vi "Remove trailing zeros.vi"(11 "Number":string) -> (3 "Number with trainlg zeros removed":string)   [LabVIEW 2017, in "JSONtext.lvlib"]
uses:
  JSONtext.lvlib
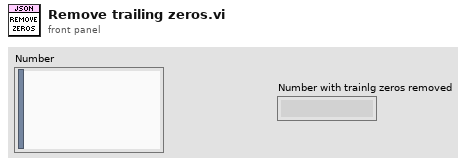
[diagram p1: front panel]
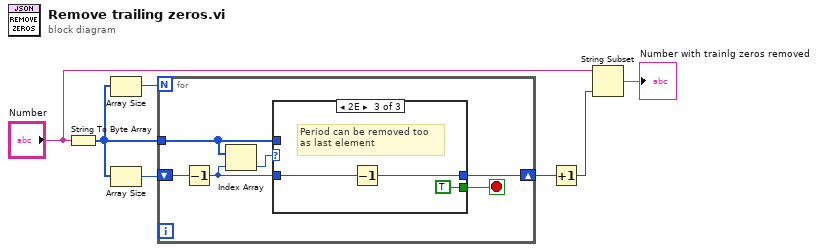
[diagram p0: block diagram]
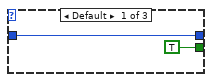
[diagram p2: hidden frame]
diagram:
  n1 = String To Byte Array(string="Number") -> (unsigned byte array=w2:u8[])
  n2 = Array Size(array=w2) -> (size(s)=w1:i32)
  n3 = Array Size(array=w2) -> (size(s)=w7:i32)
  n4 = for {
    N: w1 -> [_]
    tunnel: w2 -> [w12]
    shift-right: [w11] -> w5
    shift-left: w7 -> [w10]
    stop <- w9 stop-if-true
    n5 = Decrement(x=w10) -> (x-1=w8:i32)
    n6 = Index Array(array=w12, index=w8) -> (element=w13:u8)
    n7 = case shown="2E" w13 {
      tunnel: w12 -> [_ _ _]
      tunnel: [TRUE _ TRUE] -> w9
      tunnel: w8 -> [w14 w16 w19]
      tunnel: [w14 w16 w17] -> w11
      frame Default {
      }
      frame 48 {
      }
      frame 46 {
        # "Period can be removed too\nas last element"
        n8 = Decrement(x=w19) -> (x-1=w17:i32)
      }
    }
  }
  n9 = Increment(x=w5) -> (x+1=w4:i32)
  n10 = String Subset(string="Number", length (rest)=w4) -> (substring=→"Number with trainlg zeros removed":string)  [unwired: 1 in]
